vi "CAN Initialize FD.vi"(8 "错误输入（无错误）":errorcluster, 10 "BitrateFD":string, 11 "Channel":u16) -> (0 "错误输出":errorcluster, 1 "Channel out":u16, 2 "BitrateFD out":string, 3 "function return":u32)   [LabVIEW 2021, in "PCANBasic.lvlib"]
doc: "TPCANStatus __stdcall CAN_InitializeFD(\n TPCANHandle Channel,\n TPCANBitrateFD BitrateFD);"
uses:
  PCANBasic.lvlib
  PCANBasic.dll
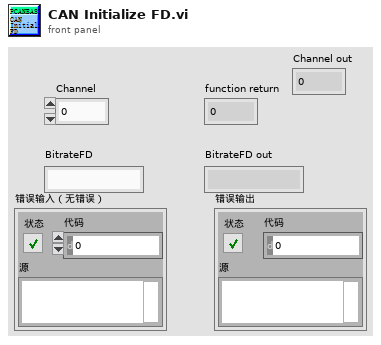
[diagram p1: front panel]
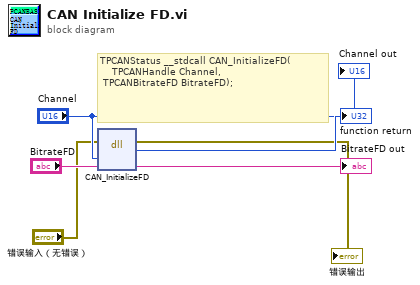
[diagram p0: block diagram]
diagram:
  # "TPCANStatus __stdcall CAN_InitializeFD(\n    TPCANHandle Channel,\n\tTPCANBitrateFD BitrateFD);"
  n1 = dll-call lib="PTH2_abs CUsersAdministrator.CH-202202160008Desktop传感器测试\tcan驱动PCANBasic.*" fn="CAN_InitializeFD"(error in="错误输入（无错误）", "Channel"="Channel", "BitrateFD"="BitrateFD") -> (error out=→"错误输出":errorcluster, "返回类型"=→"function return":u16, "BitrateFD"=→"BitrateFD out":string)  [unwired: 3 in, 1 out]
  "Channel out" <- "Channel"
